vi "SetSpeed.vi"(2 "Port Number":i8=7 min=0, 3 "Acceleration Time":u16=100 max=1000, 4 "High Speed":u32=1000 min=1 max=500000, 5 "Low Speed":u32=100 min=1 max=500000, 6 "Axis Number":u8(ring)=1) -> (0 "OK Done":bool, 1 "String Received":string)   [LabVIEW 2015]
panel:
  out "Command String":string
  # "Port Number 0=COM1"
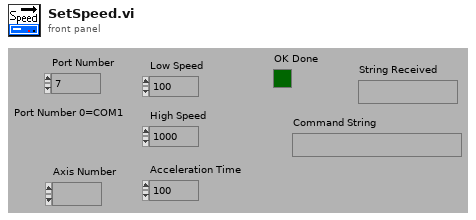
[diagram p1: front panel]
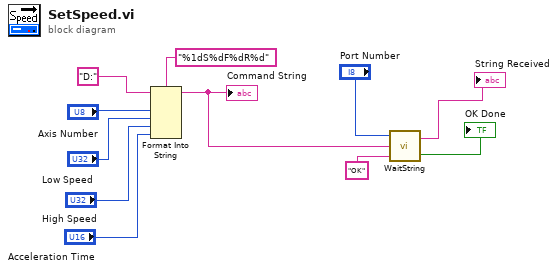
[diagram p0: block diagram]
diagram:
  n1 = Format Into String(format string="%1dS%dF%dR%d", initial string="D:", "Axis Number", "Low Speed", "High Speed", "Acceleration Time") -> (resulting string=w3:string)  [unwired: 1 in, 1 out]
  "Command String" <- w3
  n2 = call "WaitString.vi"("String to Receive"="OK", "String to Send"=w3, "PortNumber"="Port Number") -> ("OK Done"=→"OK Done":bool, "String Received"=→"String Received":string)
